vi "loopback cluster.vi"() -> ()   [LabVIEW 2013, in "Unix Pipes.lvlib"]
uses:
  Unix Pipes.lvlib
  Classes/Unix Pipe Reader/Open Pipe (reader).vi
  Classes/Unix Pipe Writer/Open Pipe (writer).vi
  Classes/Unix Pipe Reader/Close Pipe (reader).vi
  Classes/Unix Pipe Writer/Close Pipe (writer).vi
  <vilib>/NI/NI Linux RT Utilities/VIs/Public/Time/Get Clock Time (timespec).vi
  <vilib>/NI/NI Linux RT Utilities/Linux RT Utilities.lvlib
  Classes/Unix Pipe Writer/Unix Pipe Writer.lvclass
  Classes/Unix Pipe Reader/Unix Pipe Reader.lvclass
panel:
  out "stop":bool
  out "pipe already exists?":bool
  in  "stop":bool
  out "time":cluster{"sec":u64, "nsec":u64}
  out "bytes read":i32
  out "error out":errorcluster
  out "bytes written":i32
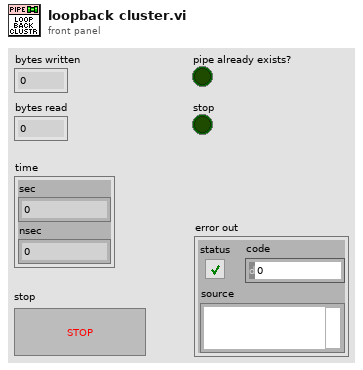
[diagram p1: front panel]
types:
  T1 = cluster{"Stop":bool, "Time":cluster{"sec":u64, "nsec":u64}}
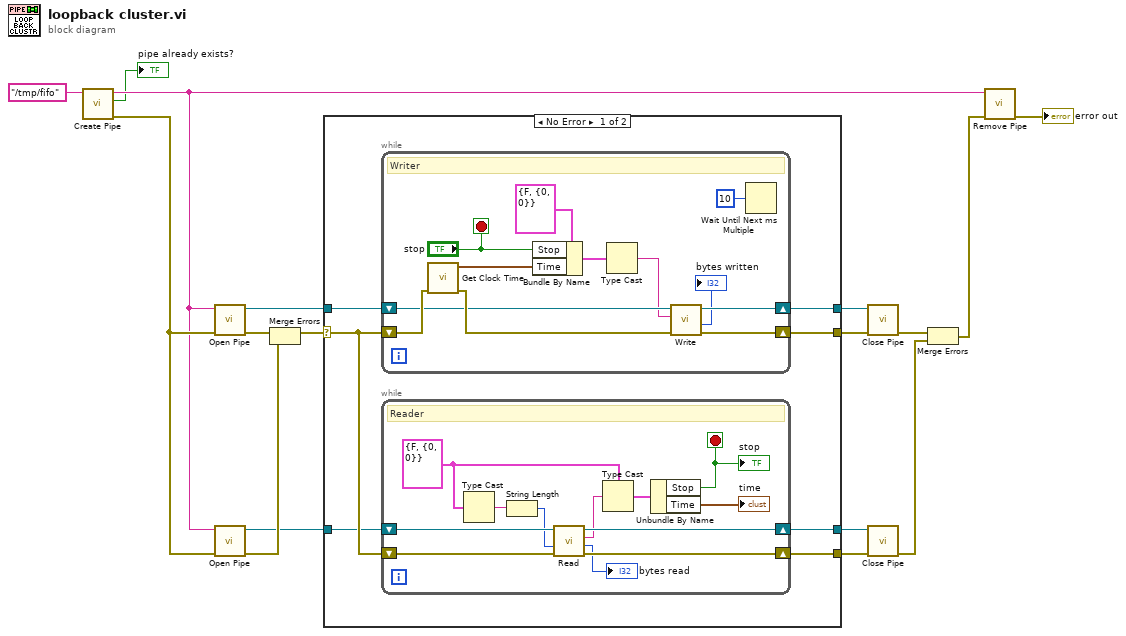
[diagram p0: block diagram]
diagram:
  n1 = call "Create Pipe.vi"("pathname in"="/tmp/fifo") -> ("error out"=w16:errorcluster, "pipe already exists?"=→"pipe already exists?":bool, "pathname out"=w15:string)  [unwired: 8 in]
  n2 = call-poly "Open Pipe.vi"("error in (no error)"=w16, "pathname in"=w15) -> ("error out"=w5:errorcluster, "pipe writer out"=w12:refnum<data-value>)  [unwired: 8 in]
  n3 = call-poly "Open Pipe.vi"("error in (no error)"=w16, "pathname in"=w15) -> ("error out"=w4:errorcluster, "pipe reader out"=w2:refnum<data-value>)  [unwired: 8 in]
  n4 = Merge Errors(w5, w4) -> (w3:errorcluster)
  n5 = case shown="No Error" w3 {
    selector: w3 -> [w19 w50]
    tunnel: w12 -> [w24 w51]
    tunnel: [w23 w51] -> w11
    tunnel: [w22 w50] -> w10
    tunnel: w2 -> [w18 w49]
    tunnel: [w21 w49] -> w9
    tunnel: [w20 w50] -> w8
    frame No Error {
      n6 = while {
        shift-right: [w47] -> w23
        shift-left: w24 -> [w41]
        shift-right: [w46] -> w22
        shift-left: w19 -> [w44]
        stop <- "stop" stop-if-true
        # "Writer"
        n7 = call-poly <vilib>:"Get Clock Time.vi"("error in (no error)"=w44) -> ("error out"=w42:errorcluster, "timespec"=w39:cluster{"sec":u64, "nsec":u64})  [unwired: 9 in]
        n8 = Bundle By Name(cluster=T1 {"Stop"=FALSE, "Time"={"sec"=0, "nsec"=0}}, "Stop"="stop", "Time"=w39) -> (w43:T1)
        n9 = Type Cast(x=w43) -> (*(type *) &x=w40:string)  [unwired: 1 in]
        n10 = call "Write.vi"("error in (no error)"=w42, "data"=w40, "pipe writer in"=w41) -> ("error out"=w46:errorcluster, "bytes written"=→"bytes written":i32, "pipe writer out"=w47:refnum<data-value>)  [unwired: 6 in]
        n11 = Wait Until Next ms Multiple(millisecond multiple=u32 10 ("wait")) -> ()  [unwired: 1 out]
      }
      n12 = while {
        shift-right: [w31] -> w21
        shift-left: w18 -> [w35]
        shift-right: [w30] -> w20
        shift-left: w19 -> [w34]
        stop <- w25 stop-if-true
        w32 = T1 {"Stop"=FALSE, "Time"={"sec"=0, "nsec"=0}}
        # "Reader"
        n13 = Type Cast(x=w32) -> (*(type *) &x=w36:string)  [unwired: 1 in]
        n14 = String Length(string=w36) -> (length=w33:i32)
        n15 = call "Read.vi"("error in (no error)"=w34, "bytes to read"=w33, "pipe reader in"=w35) -> ("error out"=w30:errorcluster, "bytes read"=→"bytes read":i32, "data"=w29:string, "pipe reader out"=w31:refnum<data-value>)  [unwired: 5 in]
        n16 = Type Cast(type=w32, x=w29) -> (*(type *) &x=w27:T1)
        n17 = Unbundle By Name(w27) -> ("Stop"=w25:bool, "Time"=→"time":cluster{"sec":u64, "nsec":u64})
        "stop" <- w25
      }
    }
    frame Error {
    }
  }
  n18 = call-poly "Close Pipe.vi"("error in (no error)"=w10, "pipe in"=w11) -> ("error out"=w7:errorcluster)  [unwired: 8 in, 1 out]
  n19 = call-poly "Close Pipe.vi"("error in (no error)"=w8, "pipe in"=w9) -> ("error out"=w6:errorcluster)  [unwired: 8 in, 1 out]
  n20 = Merge Errors(w7, w6) -> (w1:errorcluster)
  n21 = call "Remove Pipe.vi"("error in (no error)"=w1, "pathname in"=w15) -> ("error out"=→"error out":errorcluster)  [unwired: 9 in]
